vi "Self-Test.vi"() -> ()   [LabVIEW 2021, in "Ceyear.lvlib"]
doc: "Runs the instrument's self-test routine and returns the test results."
uses:
  <instrlib>/Ceyear/Ceyear.lvlib
panel:
  out "Self-Test Response":string
  out "error out":errorcluster
  out "VISA resource name out":refnum<visa-resource-name>
  in  "VISA resource name":refnum<visa-resource-name>
  in  "error in (no error)":errorcluster
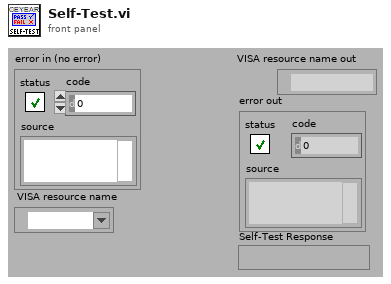
[diagram p1: front panel]
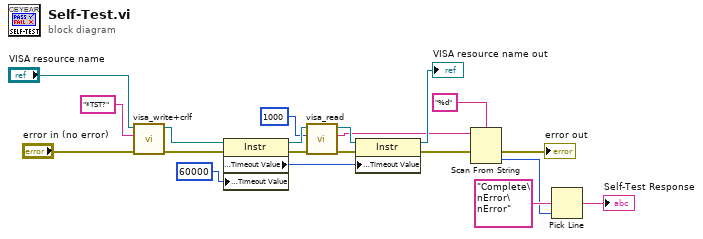
[diagram p0: block diagram]
diagram:
  n1 = call <instrlib>:"visa_write+crlf.vi"("error in (no error)"="error in (no error)", "Strings (empty)"="*TST?", "VISA resource name"="VISA resource name") -> ("error out"=w7:errorcluster, "VISA resource name out"=w8:refnum<visa-resource-name>)  [unwired: 7 in]
  n2 = property class="Instr"(reference=w8, error in=w7, "General Settings:Timeout Value"=u32 60000) -> (reference out=w6:refnum<visa-resource-name>, error out=w5:errorcluster, "General Settings:Timeout Value"=w15:u32)
  n3 = call <instrlib>:"visa_read.vi"("error in (no error)"=w5, "Byte Count (0)"=u32 1000, "VISA resource name"=w6) -> ("error out"=w1:errorcluster, "Read Data"=w2:string, "VISA resource name out"=w3:refnum<visa-resource-name>)  [unwired: 5 in, 1 out]
  n4 = property class="Instr"(reference=w3, error in=w1, "General Settings:Timeout Value"=w15) -> (reference out=→"VISA resource name out":refnum<visa-resource-name>, error out=w13:errorcluster)
  n5 = Scan From String(format string="%d", input string=w2, error in=w13) -> (error out=→"error out":errorcluster, output 1=w18:i32)  [unwired: 2 in, 2 out]
  n6 = Pick Line(multi-line string="Complete\nError\nError", line index=w18) -> (output string=→"Self-Test Response":string)  [unwired: 1 in]
